vi "Read Dependencies.vi"(8 "error in (no error)":errorcluster, 11 "Shape in":refnum<class "Shape.lvclass">) -> (0 "error out":errorcluster, 2 "Dependencies":refnum<data-value>[](array[refnum]), 3 "Shape out":refnum<class "Shape.lvclass">)   [LabVIEW 2015, in "LV Image Editor Framework.lvlib" / "Shape.lvclass"]
uses:
  Shape.lvclass
  Shape.lvclass/Shape.ctl
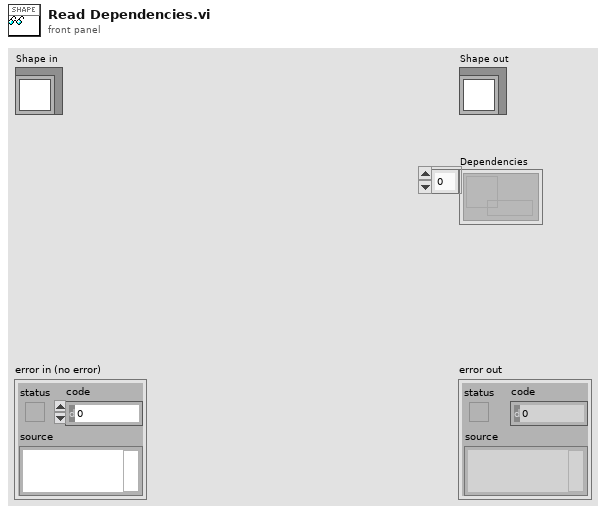
[diagram p1: front panel]
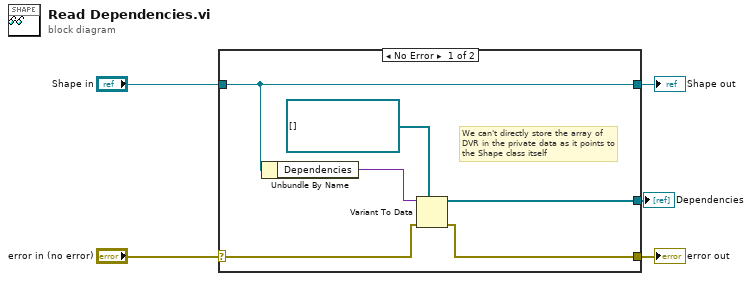
[diagram p0: block diagram]
diagram:
  n1 = case shown="No Error" "error in (no error)" {
    selector: "error in (no error)" -> [w7 w12]
    tunnel: [w6 w12] -> w4
    tunnel: [w11 w13] -> w2
    tunnel: "Shape in" -> [w11 w13]
    tunnel: [w8 _] -> w1
    frame No Error {
      # "We can't directly store the array of DVR in the private data as it points to the Shape class itself"
      n2 = Unbundle By Name(w11) -> ("Dependencies"=w10:variant)
      n3 = Variant To Data(error in=w7, type=refnum<data-value>[] [] ("Selected"), Variant=w10) -> (data=w8:refnum<data-value>[], error out=w6:errorcluster)
    }
    frame Error {
    }
  }
  "error out" <- w4
  "Shape out" <- w2
  "Dependencies" <- w1
